vi "Write ADU Packet.vi"(8 "error in":errorcluster, 9 "modbus data unit":refnum<class "Modbus Data Unit.lvclass">, 10 "isMaster (f)":bool, 11 "RTU transmission data unit in":refnum<class "RTU Data Unit.lvclass">) -> (0 "error out":errorcluster, 3 "RTU transmission data unit out":refnum<class "RTU Data Unit.lvclass">)   [LabVIEW 2021, in "RTU Data Unit.lvclass"]
uses:
  RTU Data Unit.lvclass
  D:/my_projects/projects/Algorithms/Labview/21/Modbus_v121c/Transmission Data Unit/Serial Interface/Serial Data Unit.lvclass
  D:/my_projects/projects/Algorithms/Labview/21/Modbus_v121c/Transmission Data Unit/Transmission Data Unit.lvclass
  Modbus Data Unit/Modbus Data Unit.lvclass
  Modbus Data Unit/Modbus Data Unit.lvclass/Modbus Data Unit.ctl
  Serial Interface/Serial Data Unit.lvclass/Serial Data Unit.ctl
  Transmission Data Unit.lvclass/Transmission Data Unit.ctl
  Transmission Data Unit.lvclass
  Serial Interface/Serial Data Unit.lvclass
  Network Interface/Serial Interface/SSC/Serial Shared Components.lvlib
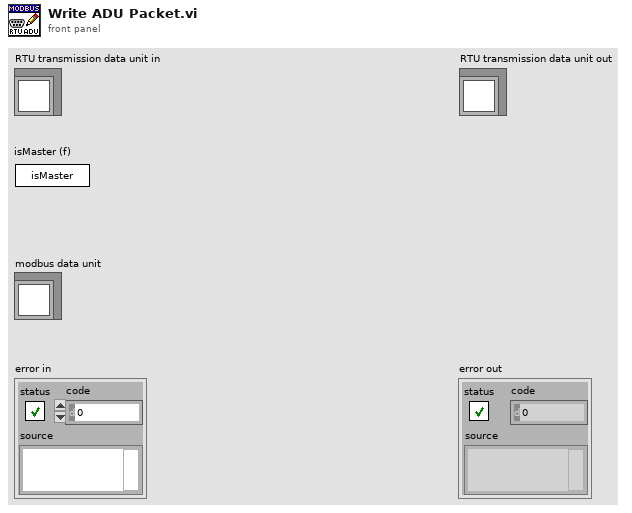
[diagram p1: front panel]
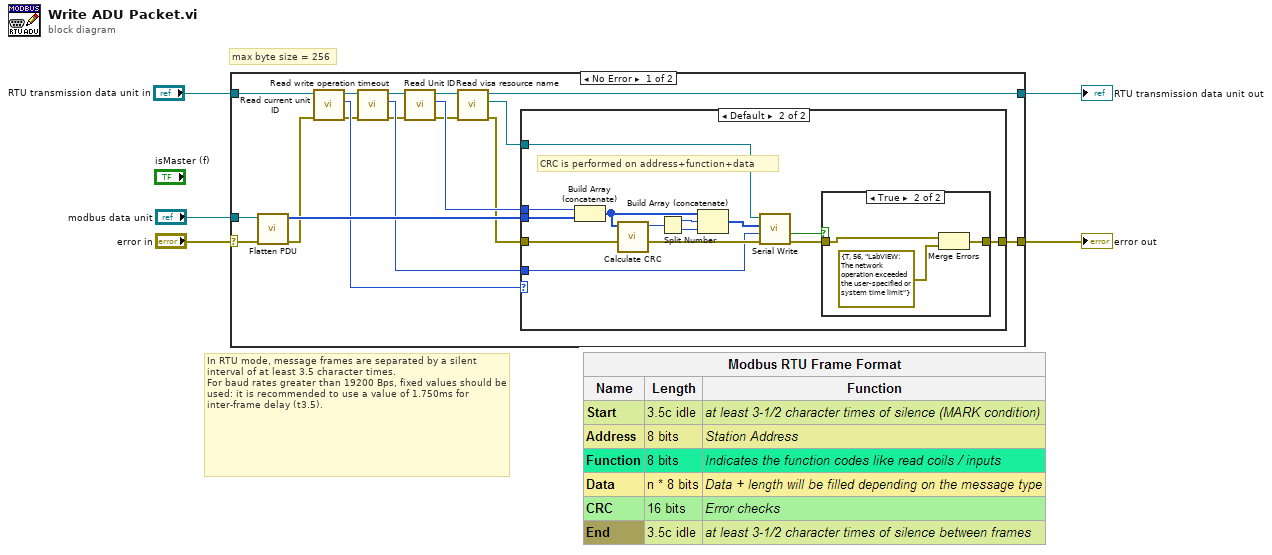
[diagram p0: block diagram]
diagram:
  # "max byte size = 256"
  # "In RTU mode, message frames are separated by a silent interval of at least 3.5 character times.\nFor baud rates greater than 19200 Bps, fixed values should be used: it is recommended to use a value of 1.750ms for inter-frame delay (t3.5)."
  n1 = case shown="No Error" "error in" {
    selector: "error in" -> [w20 w43]
    tunnel: [w21 w43] -> w1
    tunnel: "modbus data unit" -> [w23 _]
    tunnel: "RTU transmission data unit in" -> [w12 w42]
    tunnel: [w7 w42] -> w2
    frame No Error {
      n2 = call "Flatten PDU.vi"("error in"=w20, "modbus data unit in"=w23) -> ("error out"=w13:errorcluster, "Full modbus data unit"=w22:u8[])  [unwired: 8 in]
      n3 = call "Read current unit ID.vi"("error in (no error)"=w13, "Serial Data Unit in"=w12) -> ("error out"=w14:errorcluster, "request unit ID"=w19:u8, "Serial Data Unit out"=w11:refnum<class "RTU Data Unit.lvclass">)  [unwired: 7 in]
      n4 = call "Read write operation timeout.vi"("error in (no error)"=w14, "transmission data unit in"=w11) -> ("error out"=w15:errorcluster, "write operation timeout"=w18:i32, "transmission data unit out"=w16:refnum<class "RTU Data Unit.lvclass">)  [unwired: 7 in]
      n5 = call "Read Unit ID.vi"("error in"=w15, "transmission data unit in"=w16) -> ("error out"=w8:errorcluster, "unit ID"=w17:u8, "transmission data unit out"=w10:refnum<class "RTU Data Unit.lvclass">)  [unwired: 7 in]
      n6 = call "Read visa resource name.vi"("error in (no error)"=w8, "Serial Data Unit in"=w10) -> ("error out"=w6:errorcluster, "visa resource name"=w9:refnum<visa-resource-name>, "Serial Data Unit out"=w7:refnum<class "RTU Data Unit.lvclass">)  [unwired: 7 in]
      n7 = case shown="Default" w19 {
        tunnel: w22 -> [_ w37]
        tunnel: w17 -> [_ w36]
        tunnel: w6 -> [w24 w35]
        tunnel: w9 -> [_ w34]
        tunnel: [w24 w26] -> w21
        tunnel: w18 -> [_ w25]
        frame 0 {
          # "request unit ID defaults to 1. If it is 0 it was set that way. If it was set that way, this is a slave trying to respond to a broadcast"
        }
        frame Default {
          # "CRC is performed on address+function+data"
          n8 = Build Array (concatenate)(w36, w37) -> (w33:u8[])
          n9 = call "Calculate CRC.vi"("data"=w33) -> ("CRC-16"=w31:u16)  [unwired: 10 in]
          n10 = Split Number(x=w31) -> (hi(x)=w30:u8, lo(x)=w29:u8)
          n11 = Build Array (concatenate)(w33, w30, w29) -> (w32:u8[])
          n12 = call "Serial Write.vi"("error in"=w35, "timeout (ms)"=w25, "data"=w32, "Visa Resource"=w34) -> ("error out"=w27:errorcluster, "timed out?"=w28:bool)  [unwired: 6 in]
          n13 = case shown="True" w28 {
            tunnel: w27 -> [w38 w40]
            tunnel: [w38 w41] -> w26
            frame False {
            }
            frame True {
              n14 = Merge Errors(w40, errorcluster {"status"=TRUE, "code"=56, "source"="LabVIEW: The network operation exceeded the user-specified or system time limit"} ("error out")) -> (w41:errorcluster)
            }
          }
        }
      }
    }
    frame Error {
    }
  }
  "error out" <- w1
  "RTU transmission data unit out" <- w2
